vi "DuplicateClientNames.vi"() -> (3 "Multicolumn Listbox ref":refnum<vi>)   [LabVIEW 2021]
panel:
  in  "Multicolumn Listbox":i32(listbox)
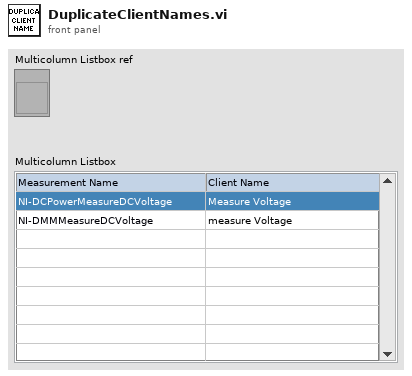
[diagram p1: front panel]
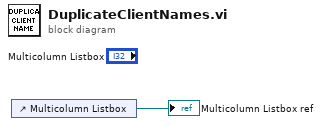
[diagram p0: block diagram]
diagram:
  n1 = control-ref of="Multicolumn Listbox"() -> (→"Multicolumn Listbox ref":refnum<vi>)
